vi "ClientSrv Runlevels Module.vi"(5 "LuaVIEW reference":T1, 7 "function index":i32) -> (15 "error out":errorcluster)   [LabVIEW 2012]
doc: "Module required by the \"runlevels.lua\" script. It assists with the configuration, starting, and stopping of runlevels."
uses:
  luaview/typedefs/t_LuaVIEW Reference.ctl
  typedefs/t_ClientSrv Runlevels Methods.ctl
  luaview/subvis/private/LuaVIEW Pull (string).vi
  luaview/subvis/private/LuaVIEW Pull (refnum).vi
  luaview/subvis/private/LuaVIEW Push (path).vi
  luaview/subvis/private/LuaVIEW Push (flat data).vi
  luaview/subvis/private/LuaVIEW Push (string).vi
  luaview/subvis/private/LuaVIEW Pull (boolean).vi
  subvis/private/glb_ClientSrv Globals.vi
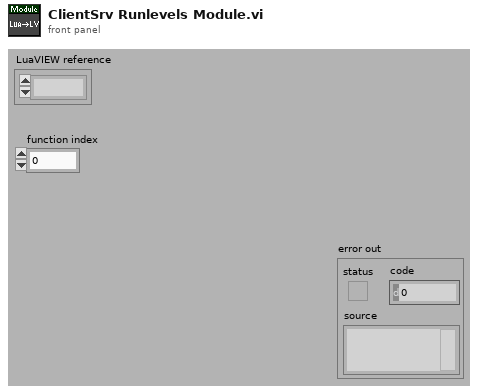
[diagram p1: front panel]
types:
  T1 = typedef "t_LuaVIEW Reference.ctl" = refnum<k1>
  T2 = enum32{"initialize", "str:path=getpath(str:lvl)", "tab:lvls=getlevels()", "str:currentlvl=getcurrent()", "setcurrent(str:lvl)", "setreboot(bool:reboot)", "cleanup()"}
  T3 = typedef "t_ClientSrv Runlevels Methods.ctl" = enum16{"initialize", "get path", "get levels", "get modes", "set current", "cleanup"}
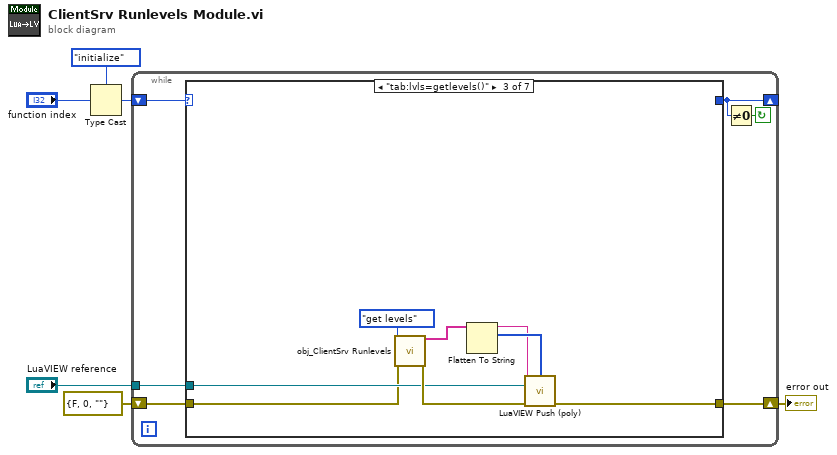
[diagram p0: block diagram]
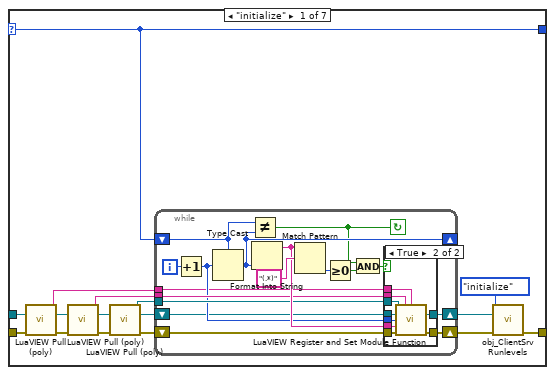
[diagram p2: hidden frame]
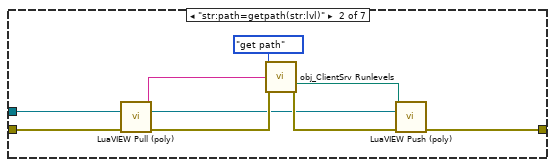
[diagram p4: hidden frame]
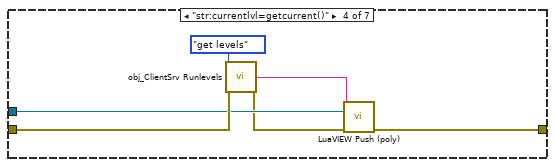
[diagram p5: hidden frame]
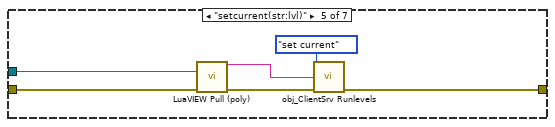
[diagram p6: hidden frame]
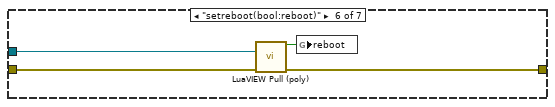
[diagram p7: hidden frame]
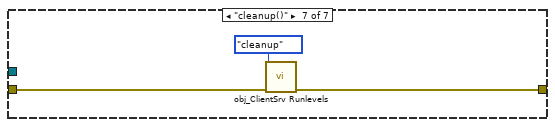
[diagram p8: hidden frame]
diagram:
  n1 = Type Cast(type=T2."initialize" ("cases"), x="function index") -> (*(type *) &x=w5:T2)
  n2 = while {
    shift-right: [w8] -> _
    shift-left: w5 -> [w12]
    shift-right: [w11] -> w6
    shift-left: errorcluster {"status"=FALSE, "code"=0, "source"=""} ("error out") -> [w10]
    tunnel: "LuaVIEW reference" -> [w9]
    stop <- w7 continue-if-true
    n3 = case shown="\"tab:lvls=getlevels()\"" w12 {
      selector: w12 -> [w19 _ _ _ _ _ _]
      tunnel: [w19 _ _ _ _ _ _] -> w8
      tunnel: w9 -> [w21 w58 w71 w75 w82 w87 _]
      tunnel: [w15 w60 w66 w77 w80 w88 w91] -> w11
      tunnel: w10 -> [w20 w65 w70 w78 w84 w89 w92]
      frame "initialize" {
        n4 = call-poly "LuaVIEW Pull (poly).vi"("LuaVIEW reference in"=w21, "error in (no error)"=w20) -> ("string"=w24:string, "LuaVIEW reference out"=w26:T1, "error out"=w25:errorcluster)  [unwired: 11 in]
        n5 = call-poly "LuaVIEW Pull (poly).vi"("LuaVIEW reference in"=w26, "error in (no error)"=w25) -> ("string"=w28:string, "LuaVIEW reference out"=w22:T1, "error out"=w23:errorcluster)  [unwired: 11 in]
        n6 = call-poly "LuaVIEW Pull (poly).vi"("LuaVIEW reference in"=w22, "error in (no error)"=w23) -> ("refnum"=w27:refnum<vi>, "LuaVIEW reference out"=w17:T1, "error out"=w18:errorcluster)  [unwired: 11 in]
        n7 = while {
          tunnel: w24 -> [w34]
          shift-right: [w42] -> w16
          shift-left: w18 -> [w43]
          shift-right: [w38] -> _
          shift-left: w19 -> [w39]
          tunnel: w28 -> [w36]
          tunnel: w27 -> [w37]
          shift-right: [w29] -> w13
          shift-left: w17 -> [w30]
          i -> [w41]
          stop <- w31 continue-if-true
          n8 = Increment(x=w41) -> (x+1=w35:i32)
          n9 = Type Cast(type=w39, x=w35) -> (*(type *) &x=w38:T2)
          n10 = Not Equal?(x=w39, y=w38) -> (x != y?=w31:bool)
          n11 = Format Into String(w38) -> (resulting string=w40:string)  [unwired: 3 in, 1 out]
          n12 = Match Pattern(string=w40, regular expression="(.*)") -> (offset past match=w44:i32)  [unwired: 1 in, 3 out]
          n13 = Greater Or Equal To 0?(x=w44) -> (x >= 0?=w33:bool)
          n14 = And(x=w31, y=w33) -> (x .and. y?=w32:bool)
          n15 = case shown="True" w32 {
            tunnel: w34 -> [_ w50]
            tunnel: w30 -> [w46 w54]
            tunnel: w35 -> [_ w55]
            tunnel: w40 -> [_ w52]
            tunnel: [w47 w56] -> w42
            tunnel: w43 -> [w47 w53]
            tunnel: w36 -> [_ w51]
            tunnel: w37 -> [_ w49]
            tunnel: [w46 w48] -> w29
            frame False {
            }
            frame True {
              n16 = call "LuaVIEW Register and Set Module Function.vi"("module refnum"=w49, "export table (set as global)"=w51, "table (set as global)"=w50, "LuaVIEW reference in"=w54, "index"=w55, "synopsis"=w52, "error in (no error)"=w53) -> ("LuaVIEW reference out"=w48:T1, "error out"=w56:errorcluster)  [unwired: 7 in]
            }
          }
        }
        n17 = call "obj_ClientSrv Runlevels.vi"("method"=t_ClientSrv_Runlevels_Methods."initialize", "LuaVIEW reference {initialize}"=w13, "error in (no error)"=w16) -> ("error out"=w15:errorcluster)  [unwired: 9 in, 3 out]
      }
      frame "str:path=getpath(str:lvl)" {
        n18 = call-poly "LuaVIEW Pull (poly).vi"("LuaVIEW reference in"=w58, "error in (no error)"=w65) -> ("string"=w61:string, "LuaVIEW reference out"=w57:T1, "error out"=w62:errorcluster)  [unwired: 11 in]
        n19 = call "obj_ClientSrv Runlevels.vi"("method"=t_ClientSrv_Runlevels_Methods."get path", "runlevel"=w61, "error in (no error)"=w62) -> ("script path"=w59:path, "error out"=w64:errorcluster)  [unwired: 9 in, 2 out]
        n20 = call-poly "LuaVIEW Push (poly).vi"("path"=w59, "LuaVIEW reference in"=w57, "error in (no error)"=w64) -> ("error out"=w60:errorcluster)  [unwired: 11 in, 1 out]
      }
      frame "tab:lvls=getlevels()" {
        n21 = call "obj_ClientSrv Runlevels.vi"("method"=t_ClientSrv_Runlevels_Methods."get levels", "error in (no error)"=w70) -> ("names"=w69:string[], "error out"=w73:errorcluster)  [unwired: 10 in, 2 out]
        n22 = Flatten To String(anything=w69) -> (data string=w67:string, type string=w68:i16[])  [unwired: 3 in, 1 out]
        n23 = call-poly "LuaVIEW Push (poly).vi"("flat data"=w67, "type descriptor"=w68, "LuaVIEW reference in"=w71, "error in (no error)"=w73) -> ("error out"=w66:errorcluster)  [unwired: 10 in, 1 out]
      }
      frame "str:currentlvl=getcurrent()" {
        n24 = call "obj_ClientSrv Runlevels.vi"("method"=t_ClientSrv_Runlevels_Methods."get levels", "error in (no error)"=w78) -> ("current"=w76:string, "error out"=w74:errorcluster)  [unwired: 10 in, 2 out]
        n25 = call-poly "LuaVIEW Push (poly).vi"("string"=w76, "LuaVIEW reference in"=w75, "error in (no error)"=w74) -> ("error out"=w77:errorcluster)  [unwired: 11 in, 1 out]
      }
      frame "setcurrent(str:lvl)" {
        n26 = call-poly "LuaVIEW Pull (poly).vi"("LuaVIEW reference in"=w82, "error in (no error)"=w84) -> ("string"=w81:string, "error out"=w83:errorcluster)  [unwired: 11 in, 1 out]
        n27 = call "obj_ClientSrv Runlevels.vi"("method"=t_ClientSrv_Runlevels_Methods."set current", "runlevel"=w81, "error in (no error)"=w83) -> ("error out"=w80:errorcluster)  [unwired: 9 in, 3 out]
      }
      frame "setreboot(bool:reboot)" {
        n28 = call-poly "LuaVIEW Pull (poly).vi"("LuaVIEW reference in"=w87, "error in (no error)"=w89) -> ("boolean"=w86:bool, "error out"=w88:errorcluster)  [unwired: 11 in, 1 out]
        n29 = global write "glb_ClientSrv Globals.vi" "reboot"(w86) -> ()
      }
      frame "cleanup()" {
        n30 = call "obj_ClientSrv Runlevels.vi"("method"=t_ClientSrv_Runlevels_Methods."cleanup", "error in (no error)"=w92) -> ("error out"=w91:errorcluster)  [unwired: 10 in, 3 out]
      }
    }
    n31 = Not Equal To 0?(x=w8) -> (x != 0?=w7:bool)
  }
  "error out" <- w6
